vi "Create Custom Device Channel Name.vi"(11 "Channel Path":string) -> (3 "CD Name":string)   [LabVIEW 2012, in "Running Average Custom Device.lvlib"]
uses:
  Running Average Custom Device.lvlib
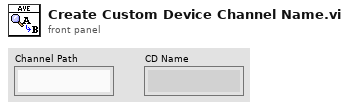
[diagram p1: front panel]
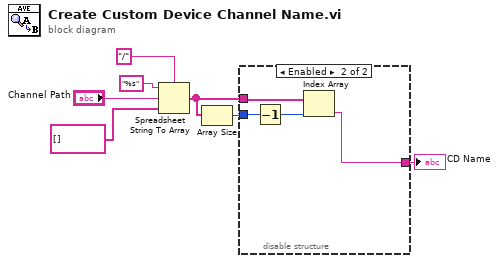
[diagram p0: block diagram]
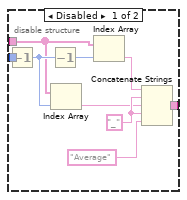
[diagram p2: hidden frame]
diagram:
  n1 = Spreadsheet String To Array(delimiter (Tab)="/", format string="%s", spreadsheet string="Channel Path", array type (2D Dbl)=string[] []) -> (array=w6:string[])
  n2 = Array Size(array=w6) -> (size(s)=w5:i32)
  n3 = disable-structure shown="Enabled" {
    disable-tunnel: [w14 w17] -> w7
    disable-tunnel: w6 -> [w10 w18]
    disable-tunnel: w5 -> [w8 w20]
    frame Disabled {
      w15 = "_"
      n4 = Decrement(x=w8) -> (x-1=w11:i32)
      n5 = Decrement(x=w11) -> (x-1=w9:i32)
      n6 = Index Array(array=w10, index=w11) -> (element=w13:string)
      n7 = Index Array(array=w10, index=w9) -> (element=w12:string)
      n8 = Concatenate Strings(w12, w15, w13, w15, "Average" ("string")) -> (w14:string)
    }
    frame Enabled {
      n9 = Decrement(x=w20) -> (x-1=w19:i32)
      n10 = Index Array(array=w18, index=w19) -> (element=w17:string)
    }
  }
  "CD Name" <- w7
